vi "ATF-DO Search channel name.vi"(10 "Data":T1={"AO config"=[], "AI config"=[], "DI config"=[], "DO config"=[], "TC config"=[], "ACC config"=[], "SG config"=[], "Strain Gauge Settings"={"poisson ratio"=0.3, "nominal gage resistance"=120.0, "gage factor"=2.08}, "Bridge Settings"={"voltage excitation value"=3.3, "voltage excitation source"=10200, "initial bridge voltage"=0.0, "lead wire resistance"=1.7, "strain configuration"=10271}, "Sample Rate"={"AI Sample Rate"=[], "AO Sample Rate"=[], "DI Sample Rate"=[], "TC Sample Rate"=[], "DO Sample Rate"=[], "SG Sample Rate"=[], "ACC Sample Rate"=[]}} {"Bridge Settings"."strain configuration" items=["Full Bridge I"=10183, "Full Bridge II"=10184, "Full Bridge III"=10185, "Half Bridge I"=10188, "Half Bridge II"=10189, "Quarter Bridge I"=10271, "Quarter Bridge II"=10272]; "Bridge Settings"."voltage excitation source" items=["Internal"=10200, "External"=10167, "None"=10230]; "ACC config"."Terminal configuration" items=["default"=-1, "RSE"=10083, "NRSE"=10078, "Differential"=10106, "Pseudodifferential"=12529]; "ACC config"."Sensitivity units" items=["mVolts/g"=12509, "Volts/g"=12510]; "TC config"."type" items=["J"=10072, "K"=10073, "N"=10077, "R"=10082, "S"=10085, "T"=10086, "B"=10047, "E"=10055]; "TC config"."units" items=["Deg C", "Deg F", "Kelvins", "Deg R", "From Custom Scale"]}) -> ()   [LabVIEW 2022 SP3]
uses:
  Controls/SeCrTs-Config.ctl
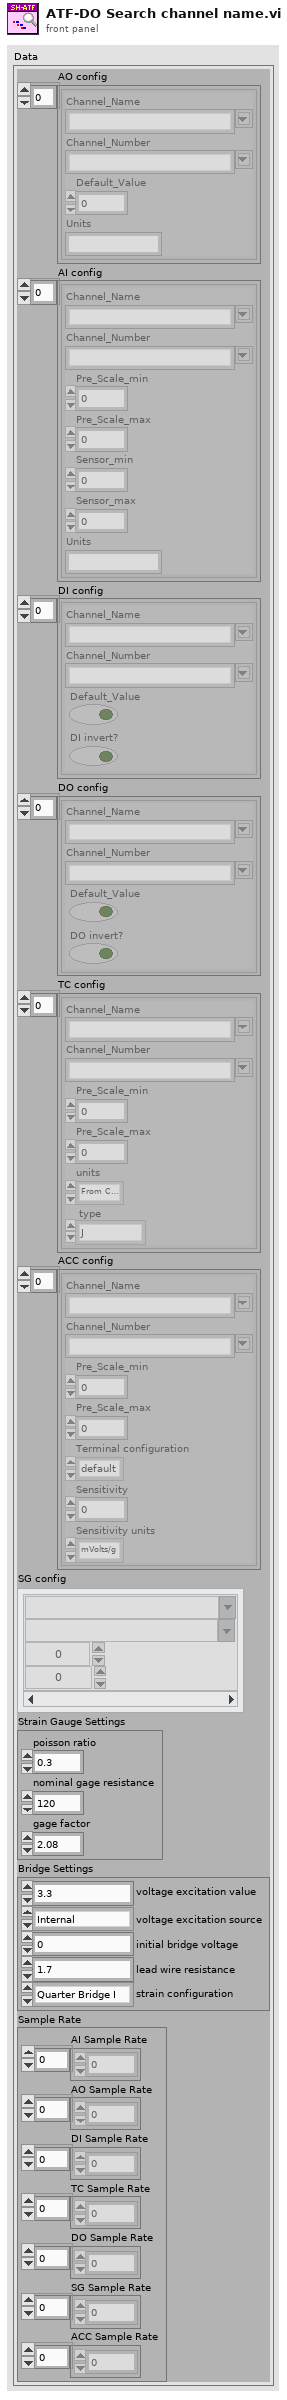
[diagram p1: front panel]
types:
  T1 = typedef "SeCrTs-Config.ctl" = cluster{"AO config":cluster{"Channel_Name":string, "Channel_Number":string, "Default_Value":dbl, "Units":string}[], "AI config":cluster{"Channel_Name":string, "Channel_Number":string, "Pre_Scale_min":dbl, "Pre_Scale_max":dbl, "Sensor_min":dbl, "Sensor_max":dbl, "Units":string}[], "DI config":cluster{"Channel_Name":string, "Channel_Number":string, "Default_Value":bool, "DI invert?":bool}[], "DO config":cluster{"Channel_Name":string, "Channel_Number":string, "Default_Value":bool, "DO invert?":bool}[], "TC config":cluster{"Channel_Name":string, "Channel_Number":string, "Pre_Scale_min":dbl, "Pre_Scale_max":dbl, "units":i32, " type":i32}[], "ACC config":cluster{"Channel_Name":string, "Channel_Number":string, "Pre_Scale_min":dbl, "Pre_Scale_max":dbl, "Terminal configuration":i32, "Sensitivity":dbl, "Sensitivity units":i32}[], "SG config":cluster{"Channel_Name":string, "Channel_Number":string, "Pre_Scale_min":dbl, "Pre_Scale_max":dbl}[], "Strain Gauge Settings":cluster{"poisson ratio":dbl, "nominal gage resistance":dbl, "gage factor":dbl}, "Bridge Settings":cluster{"voltage excitation value":dbl, "voltage excitation source":i32, "initial bridge voltage":dbl, "lead wire resistance":dbl, "strain configuration":i32}, "Sample Rate":cluster{"AI Sample Rate":dbl[], "AO Sample Rate":dbl[], "DI Sample Rate":dbl[], "TC Sample Rate":dbl[], "DO Sample Rate":dbl[], "SG Sample Rate":dbl[], "ACC Sample Rate":dbl[]}}
  T2 = cluster{"Channel_Name":string, "Channel_Number":string, "Default_Value":bool, "DO invert?":bool}[]
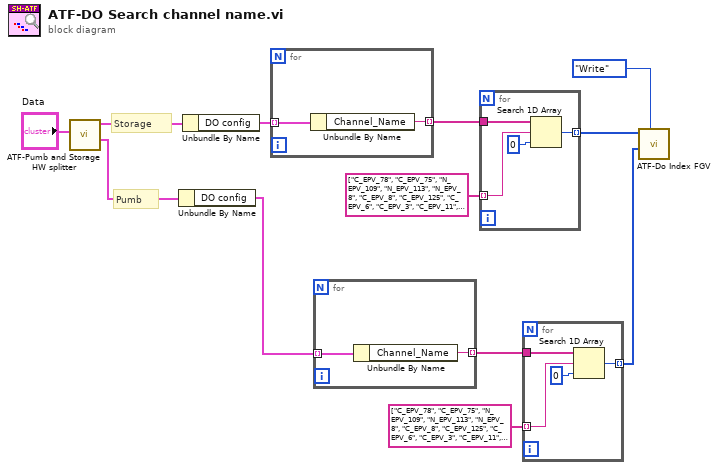
[diagram p0: block diagram]
diagram:
  # "Pumb"
  # "Storage"
  n1 = call "ATF-Pumb and Storage HW splitter.vi"("data"="Data") -> ("Pumb HW"=w5:T1, "Storage HW"=w7:T1)  [unwired: 9 in]
  n2 = Unbundle By Name(w5) -> ("DO config"=w2:T2)
  n3 = Unbundle By Name(w7) -> ("DO config"=w6:T2)
  n4 = for {
    tunnel: [w14] -> w12 mode=indexing
    tunnel: w6 -> [w13] mode=indexing
    n5 = Unbundle By Name(w13) -> ("Channel_Name"=w14:string)
  }
  n6 = for {
    tunnel: [w16] -> w3 mode=indexing
    tunnel: w2 -> [w15] mode=indexing
    n7 = Unbundle By Name(w15) -> ("Channel_Name"=w16:string)
  }
  n8 = for {
    tunnel: w12 -> [w20]
    tunnel: string[] ["C_EPV_78", "C_EPV_75", "N_EPV_109", "N_EPV_113", "N_EPV_8", "C_EPV_8", "C_EPV_125", "C_EPV_6", "C_EPV_3", "C_EPV_11", "N_EPV_190", "C_EPV_14", "C_EPV_13", "N_EPV_128", "N_EPV_150", "F_EPV_41", "N_EPV_157", "F_EPV_43", "F_EPV_38", "F_EPV_45", "N_EPV_72", "F_EPV_175", "N_EPV_138", "G_EPV_69", "M_EPV_90", "N_EPV_185"] ("Array") -> [w19] mode=indexing
    tunnel: [w17] -> w10 mode=indexing
    n9 = Search 1D Array(1D array=w20, element=w19, start index (0)=0) -> (index of element=w17:i32)
  }
  n10 = for {
    tunnel: w3 -> [w24]
    tunnel: string[] ["C_EPV_78", "C_EPV_75", "N_EPV_109", "N_EPV_113", "N_EPV_8", "C_EPV_8", "C_EPV_125", "C_EPV_6", "C_EPV_3", "C_EPV_11", "N_EPV_190", "C_EPV_14", "C_EPV_13", "N_EPV_128", "N_EPV_150", "F_EPV_41", "N_EPV_157", "F_EPV_43", "F_EPV_38", "F_EPV_45", "N_EPV_72", "F_EPV_175", "N_EPV_138", "G_EPV_69", "M_EPV_90", "N_EPV_185"] ("Array") -> [w23] mode=indexing
    tunnel: [w21] -> w1 mode=indexing
    n11 = Search 1D Array(1D array=w24, element=w23, start index (0)=0) -> (index of element=w21:i32)
  }
  n12 = call "ATF-Do Index FGV.vi"("State"=enum16{"Write", "Read"}."Write", "Pumb index"=w1, "Storage index"=w10) -> ()  [unwired: 7 in, 2 out]
